vi "Degrees to Encoder Counts.vi"(9 "Post-Shaft Gear Ratio":dbl=1.0, 11 "Degrees":dbl) -> (3 "Encoder Counts":dbl)   [LabVIEW 2015]
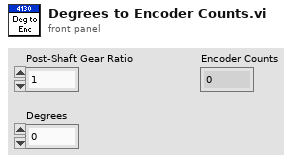
[diagram p1: front panel]
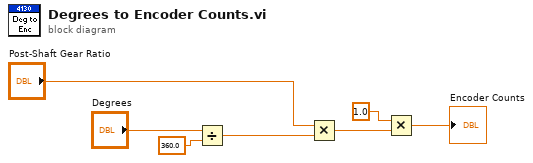
[diagram p0: block diagram]
diagram:
  n1 = Divide(x="Degrees", y=360.0) -> (x/y=w2:dbl)
  n2 = Multiply(x="Post-Shaft Gear Ratio", y=w2) -> (x*y=w4:dbl)
  n3 = Multiply(x=1.0, y=w4) -> (x*y=→"Encoder Counts":dbl)
